vi "Matrix_CommandsGlobal.vi"() -> ()   [LabVIEW 2018, in "Switching.lvclass"]
uses:
  Switching.lvclass
panel:
  in  "Pickering Matrix GPIB Setup":T1={"Matrix address"="1", "Instrument name"="Pickering Matrix", "Instrument type"=2, "Command \"Matrix Reset\""="areset %s", "Command \"Connect Matrix Channels\""="mclose %s,%d,%d", "Command \"Disconnect Matrix Channels\""="mopen %s,%d,%d"} {"Instrument type" items=["Supply", "LCR", "Switching"]}
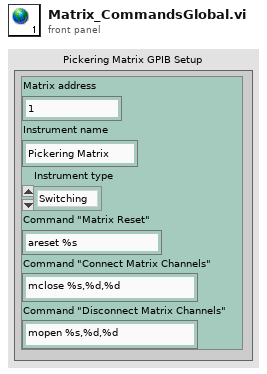
[diagram p1: front panel]
types:
  T1 = cluster{"Matrix address":string, "Instrument name":string, "Instrument type":u16, "Command \"Matrix Reset\"":string, "Command \"Connect Matrix Channels\"":string, "Command \"Disconnect Matrix Channels\"":string}
diagram:
